vi "Pre Build.vi"   [LabVIEW 2024, in "Sift Client.lvlib"]
uses:
  Sift Client.lvlib
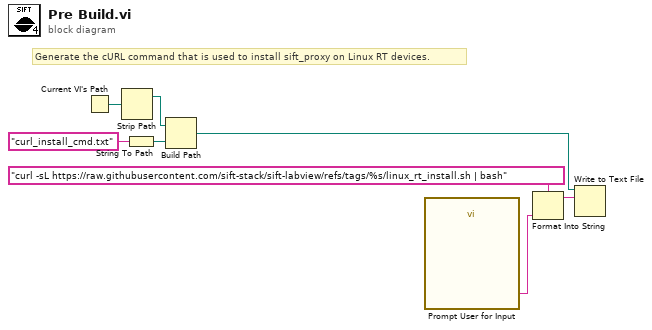
[diagram p0: block diagram]
diagram:
  # "Generate the cURL command that is used to install sift_proxy on Linux RT devices."
  n1 = Current VI's Path() -> (path=w3:path)
  n2 = Strip Path(path=w3) -> (stripped path=w2:path)  [unwired: 1 out]
  n3 = String To Path(string="curl_install_cmd.txt") -> (path=w4:path)
  n4 = Build Path(base path=w2, name or relative path=w4) -> (appended path=w1:path)
  n5 = call "Prompt User for Input"() -> ("Git Tag"=w7:string)  [unwired: 17 in, 2 out]
  n6 = Format Into String(format string="curl -sL https://raw.githubusercontent.com/sift-stack/sift-labview/refs/tags/%s/linux_rt_install.sh | bash", w7) -> (resulting string=w6:string)  [unwired: 2 in, 1 out]
  n7 = Write to Text File(file (use dialog)=w1, text=w6) -> ()  [unwired: 2 in, 3 out]
